vi "导轨控制.vi"(7 "Enum":T1(ring), 8 "error in":errorcluster, 10 "write buffer":string, 11 "转盘导轨串口":refnum<visa-resource-name>="COM61") -> (0 "error out":errorcluster, 1 "position":i32, 2 "read buffer":string)   [LabVIEW 2016]
uses:
  <vilib>/Instr/_visa.llb/VISA Flush IO Buffer Mask.ctl
  <vilib>/Instr/_visa.llb/VISA Configure Serial Port (Instr).vi
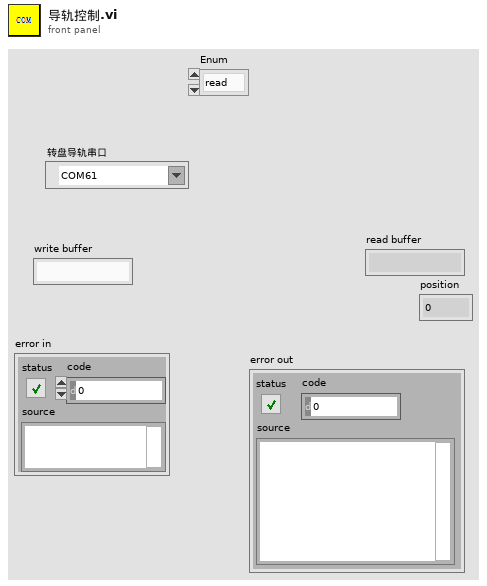
[diagram p1: front panel]
types:
  T1 = enum16{"read", "write", "release", "initial", "position calibration"}
  T2 = typedef "VISA Flush IO Buffer Mask.ctl" = u16
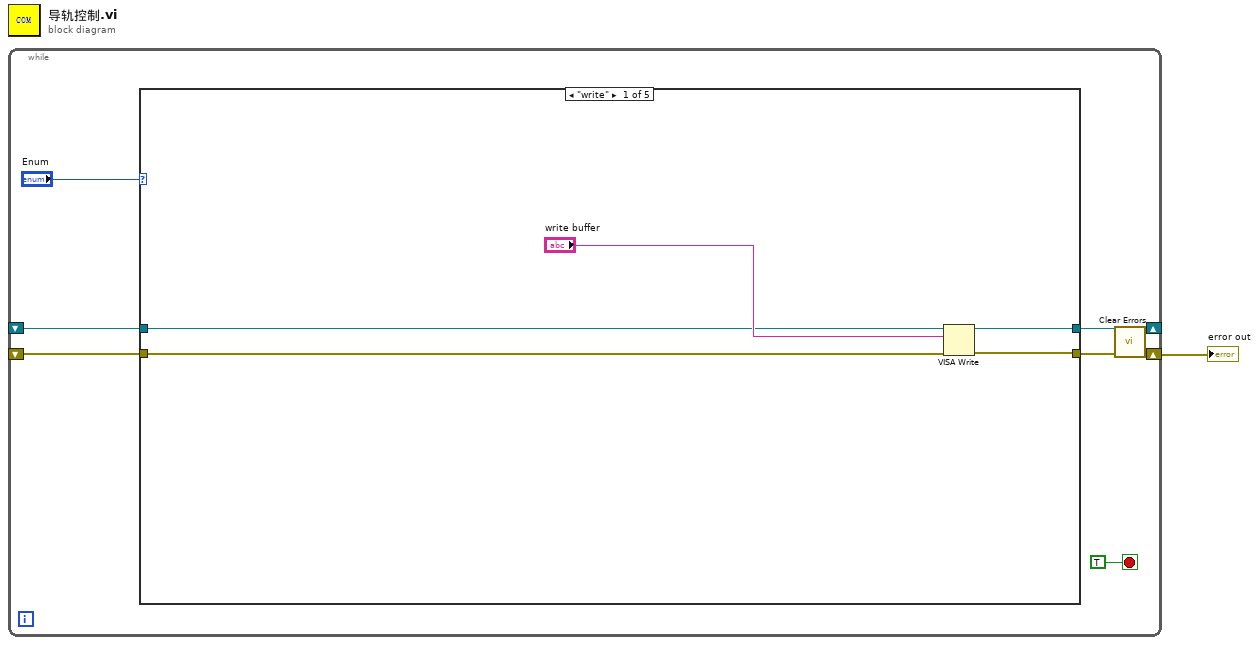
[diagram p0: block diagram]
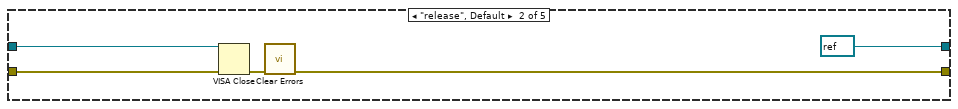
[diagram p2: hidden frame]
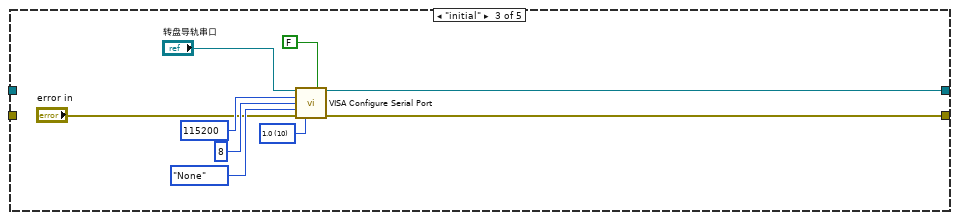
[diagram p3: hidden frame]
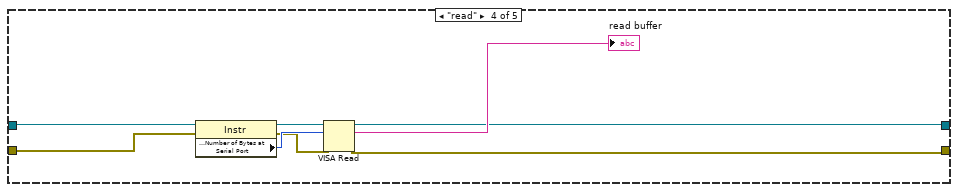
[diagram p4: hidden frame]
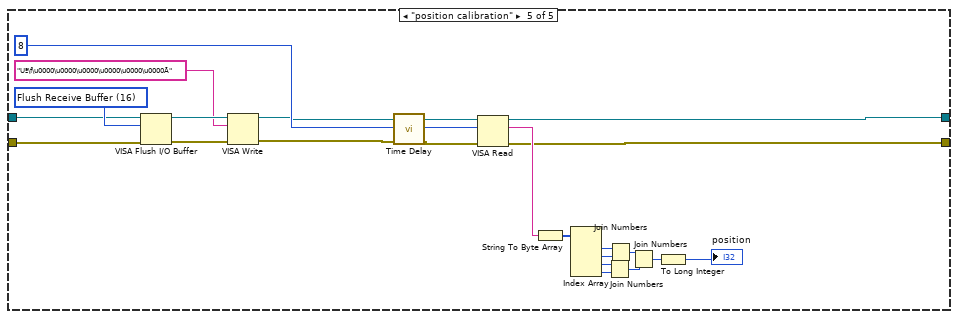
[diagram p5: hidden frame]
diagram:
  n1 = while {
    shift-right: [w2] -> w1
    shift-left: _ -> [w8]
    shift-right: [w7] -> _
    shift-left: _ -> [w6]
    stop <- TRUE stop-if-true
    n2 = case shown="\"write\"" "Enum" {
      tunnel: w8 -> [w13 w17 _ w30 w38]
      tunnel: [w12 w16 w22 w35 w36] -> w3
      tunnel: [w9 refnum<visa-resource-name> refnum ("转盘导轨串口 2") w19 w28 w37] -> w7
      tunnel: w6 -> [w10 w15 _ w29 w39]
      frame "write" {
        n3 = VISA Write(VISA resource name=w10, write buffer="write buffer", error in (no error)=w13) -> (VISA resource name out=w9:refnum<visa-resource-name>, error out=w12:errorcluster)  [unwired: 1 out]
      }
      frame "release", Default {
        n4 = VISA Close(VISA resource name=w15, error in (no error)=w17) -> (error out=w18:errorcluster)
        n5 = call <vilib>:"Clear Errors.vi"("error in (no error)"=w18) -> ("error out"=w16:errorcluster)  [unwired: 5 in, 1 out]
      }
      frame "initial" {
        w27 = u16 10 items=["1.0"=10, "1.5"=15, "2.0"=20] ("stop bits (10: 1 bit)")
        n6 = call-poly "VISA Configure Serial Port"("VISA resource name"="转盘导轨串口", "Enable Termination\nChar (T)"=FALSE ("Enable Termination\nChar (T)"), "baud rate (9600)"=u32 115200, "data bits (8)"=u16 8, "parity (0:none)"=enum16{"None", "Odd", "Even", "Mark", "Space"}."None", "error in (no error)"="error in", "stop bits (10: 1 bit)"=w27) -> ("VISA resource name out"=w19:refnum<visa-resource-name>, "error out"=w22:errorcluster)  [unwired: 7 in]
      }
      frame "read" {
        n7 = property class="Instr"(reference=w29, error in=w30) -> (reference out=w32:refnum<visa-resource-name>, error out=w31:errorcluster, "Serial Settings:Number of Bytes at Serial Port"=w33:u32)
        n8 = VISA Read(VISA resource name=w32, byte count=w33, error in (no error)=w31) -> (VISA resource name out=w28:refnum<visa-resource-name>, read buffer=→"read buffer":string, error out=w35:errorcluster)  [unwired: 1 out]
      }
      frame "position calibration" {
        w53 = T2 16 items=["Flush Receive Buffer"=16, "Write Transmit Buffer to Device"=32, "Flush Receive Buffer (No I/O)"=64, "Flush Transmit Buffer"=128] ("Mask")
        n9 = VISA Flush I/O Buffer(VISA resource name=w39, mask (16)=w53, error in (no error)=w38) -> (VISA resource name out=w54:refnum<visa-resource-name>, error out=w55:errorcluster)
        n10 = VISA Write(VISA resource name=w54, write buffer="Uª\f\u0000\u0000\u0000\u0000\u0000\u0000Ã", error in (no error)=w55) -> (VISA resource name out=w41:refnum<visa-resource-name>, error out=w56:errorcluster)  [unwired: 1 out]
        n11 = call "Time Delay"("error in (no error)"=w56) -> ("error out"=w57:errorcluster)  [unwired: 10 in]
        n12 = VISA Read(VISA resource name=w41, byte count=u32 8, error in (no error)=w57) -> (VISA resource name out=w37:refnum<visa-resource-name>, read buffer=w43:string, error out=w36:errorcluster)  [unwired: 1 out]
        n13 = String To Byte Array(string=w43) -> (unsigned byte array=w46:u8[])
        n14 = Index Array(array=w46) -> (element #1=w44:u8, element #2=w45:u8, element #3=w47:u8, element #4=w48:u8)  [unwired: 4 in]
        n15 = Join Numbers(hi=w47, lo=w48) -> ((hi.lo)=w50:u16)
        n16 = Join Numbers(hi=w44, lo=w45) -> ((hi.lo)=w49:u16)
        n17 = Join Numbers(hi=w49, lo=w50) -> ((hi.lo)=w51:u32)
        n18 = To Long Integer(number=w51) -> (32bit integer=→"position":i32)
      }
    }
    n19 = call <vilib>:"Clear Errors.vi"("error in (no error)"=w3) -> ("error out"=w2:errorcluster)  [unwired: 5 in, 1 out]
  }
  "error out" <- w1
